vi "Glyph from Codepoint.vi"(7 "DPI (75)":u32=75, 8 "error in (no error)":errorcluster, 9 "Size":sgl=16.0, 10 "codepoint":u32, 11 "face ref":i64) -> (0 "error out":errorcluster, 2 "glyph ref out":i64, 3 "face ref out":i64)   [LabVIEW 2023, in "Freetype Drawer.lvlib" / "Freetype Drawer.lvclass"]
uses:
  Freetype Drawer.lvclass
  Freetype Drawer.lvclass/Freetype Drawer.ctl
  Freetype Drawer.lvlib
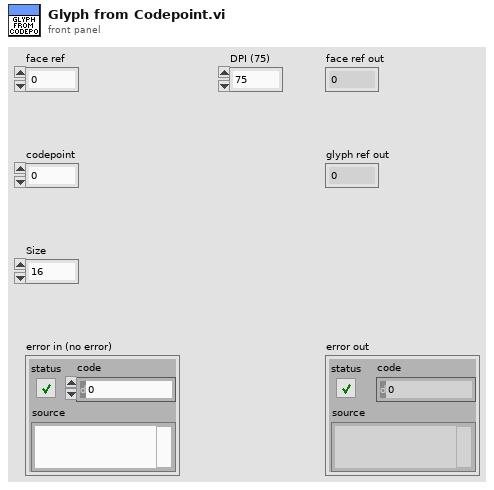
[diagram p1: front panel]
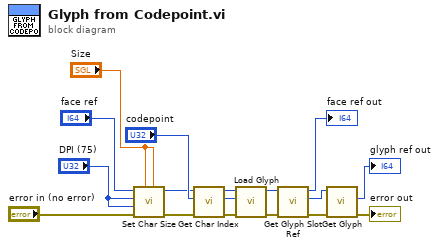
[diagram p0: block diagram]
diagram:
  n1 = call "Set Char Size.vi"("widh (same as height)"="Size", "height"="Size", "error in (no error)"="error in (no error)", "v_res"="DPI (75)", "h_res"="DPI (75)", "face in"="face ref") -> ("error out"=w4:errorcluster, "face out"=w6:i64)  [unwired: 4 in]
  n2 = call "Get Char Index.vi"("error in (no error)"=w4, "charcode"="codepoint", "face"=w6) -> ("error out"=w5:errorcluster, "index"=w8:u32, "face 2"=w7:i64)  [unwired: 6 in]
  n3 = call "Load Glyph.vi"("error in (no error)"=w5, "glyph_index"=w8, "face in"=w7) -> ("error out"=w2:errorcluster, "face out"=w3:i64)  [unwired: 7 in]
  n4 = call "Get Glyph Slot Ref.vi"("error in (no error)"=w2, "face in"=w3) -> ("error out"=w12:errorcluster, "glyph slot ref"=w11:i64, "face out"=→"face ref out":i64)  [unwired: 7 in]
  n5 = call "Get Glyph.vi"("error in (no error)"=w12, "glyph slot ref in"=w11) -> ("error out"=→"error out":errorcluster, "glyph ref out"=→"glyph ref out":i64)  [unwired: 7 in, 1 out]
